vi "Configure Level.vi"(4 "Manual Attenuation (30 dB)":dbl=30.0, 5 "Reference Level Offset (0 dB)":dbl, 6 "Auto Attenuation (T: Enable)":bool=TRUE, 7 "Reference Level (0)":dbl, 8 "error in (no error)":errorcluster, 9 "Input Impedance (0: 50 ohms)":u16(ring) items=["50", "75"], 10 "Amplitude Units (0: dBm)":u16(ring) items=["dBm", "dBV", "dBmV", "dBuV", "Volts", "Watts"], 11 "VISA resource name":refnum<visa-resource-name>) -> (0 "error out":errorcluster, 3 "VISA resource name out":refnum<visa-resource-name>)   [LabVIEW 2013, in "Template - Spectrum Analyzer.lvlib"]
doc: "Configures the vertical settings of the spectrum analyzer."
uses:
  <instrlib>/_Template - Spectrum Analyzer/Template - Spectrum Analyzer.lvlib
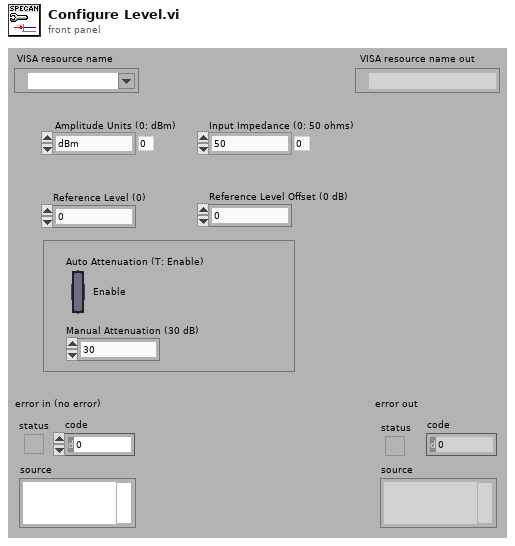
[diagram p1: front panel]
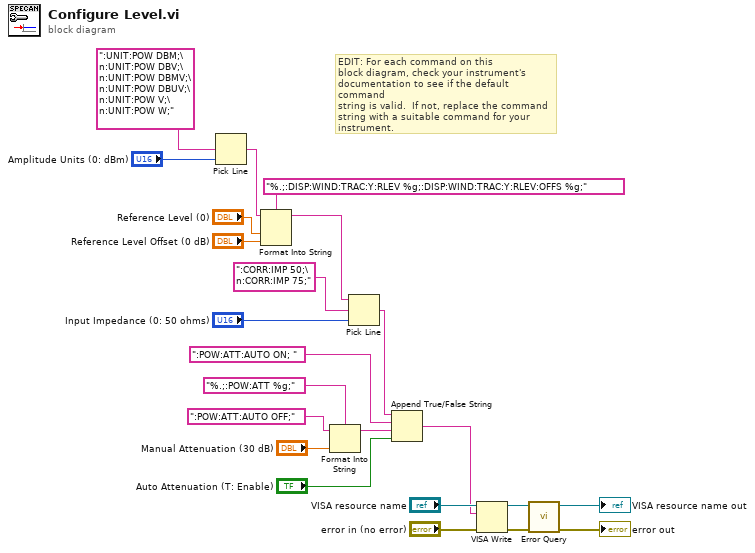
[diagram p0: block diagram]
diagram:
  # "EDIT: For each command on this\nblock diagram, check your instrument's\ndocumentation to see if the default command\nstring is valid.  If not, replace the command\nstring with a suitable command for your\ninstrument."
  n1 = Pick Line(multi-line string=":UNIT:POW DBM;\n:UNIT:POW DBV;\n:UNIT:POW DBMV;\n:UNIT:POW DBUV;\n:UNIT:POW V;\n:UNIT:POW W;", line index="Amplitude Units (0: dBm)") -> (output string=w2:string)  [unwired: 1 in]
  n2 = Format Into String(format string="%.;:DISP:WIND:TRAC:Y:RLEV %g;:DISP:WIND:TRAC:Y:RLEV:OFFS %g;", initial string=w2, "Reference Level (0)", "Reference Level Offset (0 dB)") -> (resulting string=w9:string)  [unwired: 1 in, 1 out]
  n3 = Format Into String(format string="%.;:POW:ATT %g;", initial string=":POW:ATT:AUTO OFF;" ("string (\"\")"), "Manual Attenuation (30 dB)") -> (resulting string=w14:string)  [unwired: 1 in, 1 out]
  n4 = Pick Line(string ("")=w9, multi-line string=":CORR:IMP 50;\n:CORR:IMP 75;", line index="Input Impedance (0: 50 ohms)") -> (output string=w1:string)
  n5 = Append True/False String(1:"Auto Attenuation (T: Enable)", 2:w14, 3:":POW:ATT:AUTO ON; " ("string (\"\")"), 4:w1) -> (0:w8:string)
  n6 = VISA Write(VISA resource name="VISA resource name", write buffer=w8, error in (no error)="error in (no error)") -> (VISA resource name out=w6:refnum<visa-resource-name>, error out=w4:errorcluster)  [unwired: 1 out]
  n7 = call <instrlib>:"Error Query.vi"("error in (no error)"=w4, "VISA resource name"=w6) -> ("error out"=→"error out":errorcluster, "VISA resource name out"=→"VISA resource name out":refnum<visa-resource-name>)  [unwired: 6 in, 2 out]
